vi "Initialize.vi"(8 "error in (no error)":errorcluster, 9 "transceiver settings":T1, 10 "Transfer Groups Configurations":T2[](array[typedef]) {"Transfers"."channel configurations"."buffer offset" format="%d bytes"}, 11 "MockTransceiver in":refnum<class "MockTransceiver.lvclass">) -> (0 "error out":errorcluster, 3 "MockTransceiver out":refnum<class "MockTransceiver.lvclass">)   [LabVIEW 2017, in "MockTransceiver.lvclass"]
uses:
  MockTransceiver.lvclass
  Configuration/Public/Controls/DSF Engine Transfer Group Configuration.ctl
  Configuration/Public/Controls/DSF Direction.ctl
  Configuration/Public/Controls/DSF Timing Info.ctl
  Configuration/Public/Controls/DSF Engine Transfer Configuration.ctl
  Configuration/Public/Controls/DSF Byte Order.ctl
  Configuration/Public/Controls/DSF Engine Channel Configuration.ctl
  Configuration/Public/Controls/DSF Data Type.ctl
  Configuration/Public/Controls/DSF Settings Info.ctl
  MockTransceiver.lvclass/MockTransceiver.ctl
  Engine/Classes/Transceiver/Transceiver.lvclass
  DSF Core.lvlib
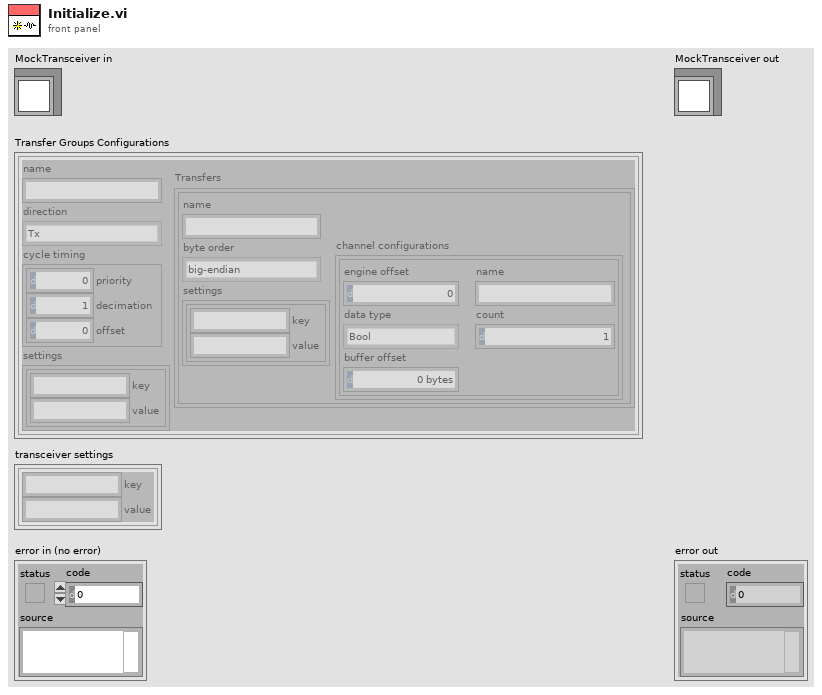
[diagram p1: front panel]
types:
  T1 = typedef "DSF Core.lvlib/DSF Settings Info.ctl" = cluster{"key":string, "value":string}[]
  T2 = typedef "DSF Core.lvlib/DSF Engine Transfer Group Configuration.ctl" = cluster{"name":string, "direction":T3, "cycle timing":T4, "Transfers":T5[], "settings":T1}
  T3 = typedef "DSF Core.lvlib/DSF Direction.ctl" = enum8{"Tx", "Rx"}
  T4 = typedef "DSF Core.lvlib/DSF Timing Info.ctl" = cluster{"priority":u64, "decimation":u64, "offset":u64}
  T5 = typedef "DSF Core.lvlib/DSF Engine Transfer Configuration.ctl" = cluster{"name":string, "byte order":T6, "channel configurations":T7[], "settings":T1}
  T6 = typedef "DSF Core.lvlib/DSF Byte Order.ctl" = enum8{"big-endian", "little-endian"}
  T7 = typedef "DSF Core.lvlib/DSF Engine Channel Configuration.ctl" = cluster{"engine offset":u64, "name":string, "data type":T8, "count":u64, "buffer offset":u64}
  T8 = typedef "DSF Core.lvlib/DSF Data Type.ctl" = enum8{"Bool", "SGL", "DBL", "I8", "I16", "I32", "I64", "U8", "U16", "U32", "U64"}
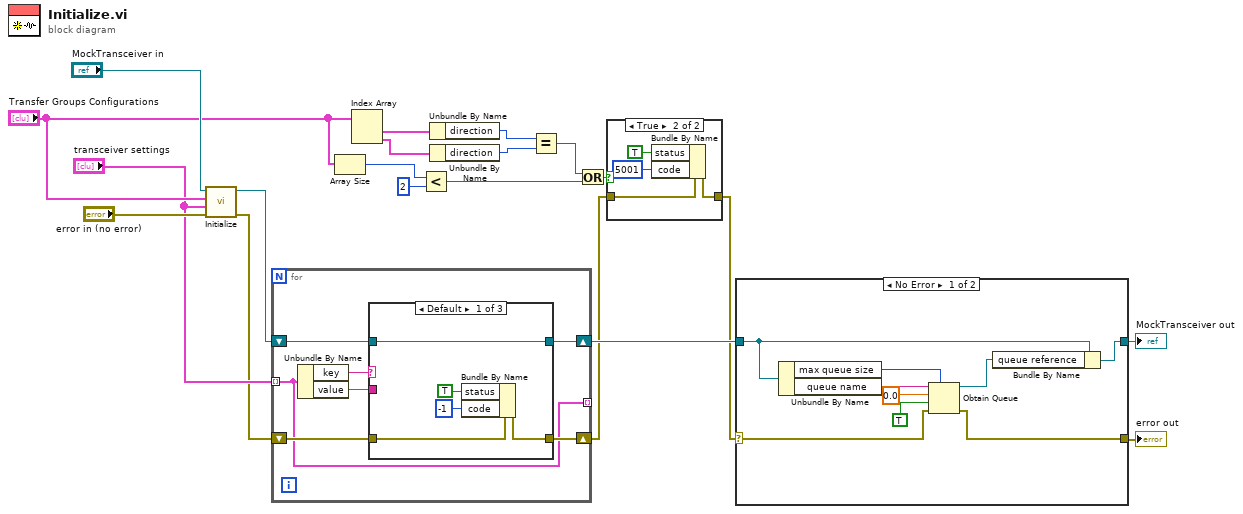
[diagram p0: block diagram]
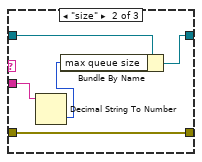
[diagram p4: hidden frame]
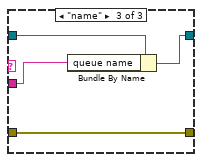
[diagram p5: hidden frame]
diagram:
  n1 = call-parent "Initialize.vi"("error in (no error)"="error in (no error)", "transceiver settings"="transceiver settings", "Transfer Groups Configurations"="Transfer Groups Configurations", "Transceiver in"="MockTransceiver in") -> ("error out"=w2:errorcluster, "Transceiver out"=w4:refnum<class "MockTransceiver.lvclass">)  [unwired: 6 in]
  n2 = for {
    tunnel: "transceiver settings" -> [w21] mode=indexing
    shift-right: [w24] -> w18
    shift-left: w4 -> [w25]
    shift-right: [w22] -> w9
    shift-left: w2 -> [w23]
    tunnel: [w21] -> _ mode=indexing
    n3 = Unbundle By Name(w21) -> ("key"=w27:string, "value"=w26:string)
    n4 = case shown="Default" w27 {
      tunnel: w26 -> [_ w35 w38]
      tunnel: w25 -> [w32 w37 w41]
      tunnel: [w32 w36 w40] -> w24
      tunnel: w23 -> [w31 w33 w39]
      tunnel: [w30 w33 w39] -> w22
      frame Default {
        n5 = Bundle By Name(cluster=w31, "status"=TRUE, "code"=-1) -> (w30:errorcluster)
      }
      frame "size" {
        n6 = Decimal String To Number(string=w35) -> (number=w34:i32)  [unwired: 2 in, 1 out]
        n7 = Bundle By Name(cluster=w37, "max queue size"=w34) -> (w36:refnum<class "MockTransceiver.lvclass">)
      }
      frame "name" {
        n8 = Bundle By Name(cluster=w41, "queue name"=w38) -> (w40:refnum<class "MockTransceiver.lvclass">)
      }
    }
  }
  n9 = Array Size(array="Transfer Groups Configurations") -> (size(s)=w17:i32)
  n10 = Index Array(array="Transfer Groups Configurations") -> (element #1=w15:T2, element #2=w14:T2)  [unwired: 2 in]
  n11 = Less?(x=w17, y=2) -> (x < y?=w10:bool)
  n12 = Unbundle By Name(w15) -> ("direction"=w12:T3)
  n13 = Unbundle By Name(w14) -> ("direction"=w13:T3)
  n14 = Equal?(x=w12, y=w13) -> (x = y?=w11:bool)
  n15 = Or(x=w11, y=w10) -> (x .or. y?=w7:bool)
  n16 = case shown="True" w7 {
    tunnel: w9 -> [w42 w44]
    tunnel: [w42 w43] -> w8
    frame False {
    }
    frame True {
      n17 = Bundle By Name(cluster=w44, "status"=TRUE, "code"=5001) -> (w43:errorcluster)
    }
  }
  n18 = case shown="No Error" w8 {
    selector: w8 -> [w48 w56]
    tunnel: [w51 w57] -> w5
    tunnel: w18 -> [w47 w57]
    tunnel: [w49 w56] -> w1
    frame No Error {
      n19 = Unbundle By Name(w47) -> ("max queue size"=w54:i32, "queue name"=w55:string)
      n20 = Obtain Queue(max queue size (-1, unlimited)=w54, name (unnamed)=w55, element data type=0.0, create if not found? (T)=TRUE, error in (no error)=w48) -> (queue out=w50:refnum<queue>, error out=w49:errorcluster)  [unwired: 1 out]
      n21 = Bundle By Name(cluster=w47, "queue reference"=w50) -> (w51:refnum<class "MockTransceiver.lvclass">)
    }
    frame Error {
    }
  }
  "error out" <- w1
  "MockTransceiver out" <- w5
